vi "Read Gains.vi"(8 "error in (no error)":errorcluster, 11 "Change Laser Gain CMD in":refnum<class "Change Laser Gain CMD.lvclass">) -> (0 "error out":errorcluster, 2 "Gains":cluster{"Red":dbl, "Blue":dbl}, 3 "Change Laser Gain CMD out":refnum<class "Change Laser Gain CMD.lvclass">)   [LabVIEW 2014, in "eCRDS Library.lvlib" / "Change Laser Gain CMD.lvclass"]
uses:
  Change Laser Gain CMD.lvclass
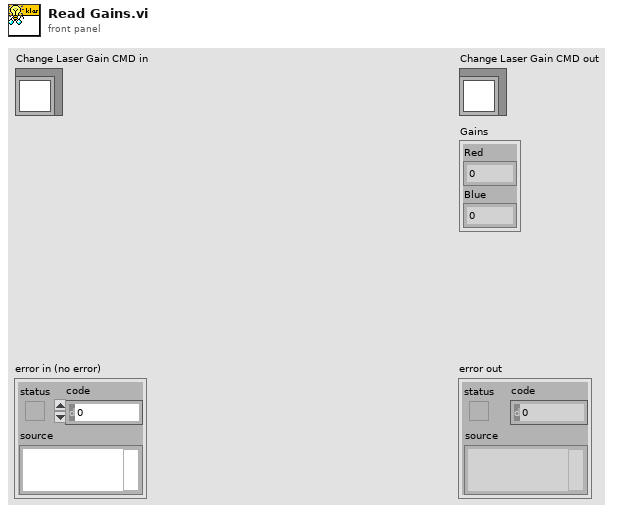
[diagram p1: front panel]
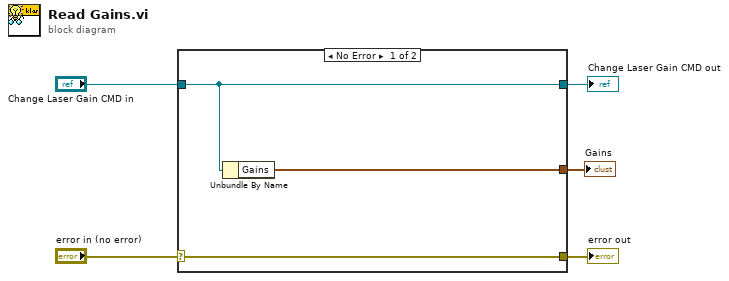
[diagram p0: block diagram]
diagram:
  n1 = case shown="No Error" "error in (no error)" {
    selector: "error in (no error)" -> [w8 w9]
    tunnel: [w8 w9] -> w4
    tunnel: [w7 w10] -> w2
    tunnel: "Change Laser Gain CMD in" -> [w7 w10]
    tunnel: [w6 _] -> w1
    frame No Error {
      n2 = Unbundle By Name(w7) -> ("Gains"=w6:cluster{"Red":dbl, "Blue":dbl})
    }
    frame Error {
    }
  }
  "error out" <- w4
  "Change Laser Gain CMD out" <- w2
  "Gains" <- w1
